vi "TargetCorrection.vi"(8 "error in (no error)":errorcluster, 9 "orientation":dbl, 10 "position(x,y)":dbl[](array[numeric]), 11 "KickToPassReceiverTactic in":refnum<class "KickToPassReceiverTactic.lvclass">) -> (0 "error out":errorcluster, 2 "TargetCorrection":dbl[](array[numeric]), 3 "KickToPassReceiverTactic out":refnum<class "KickToPassReceiverTactic.lvclass">)   [LabVIEW 2021, in "KickToPassReceiverTactic.lvclass"]
uses:
  KickToPassReceiverTactic.lvclass
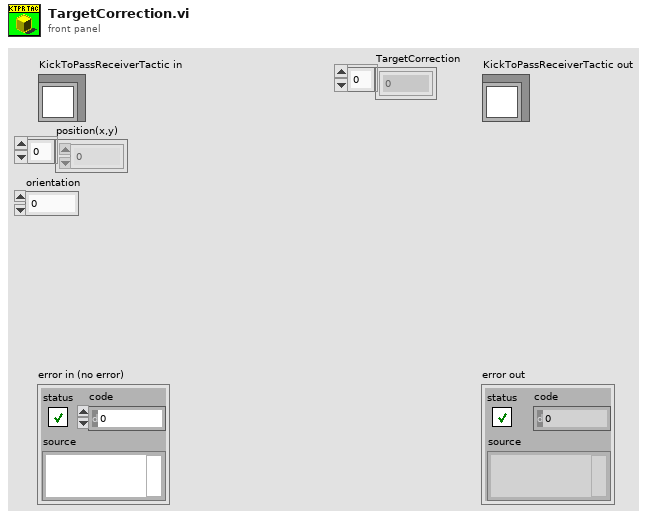
[diagram p1: front panel]
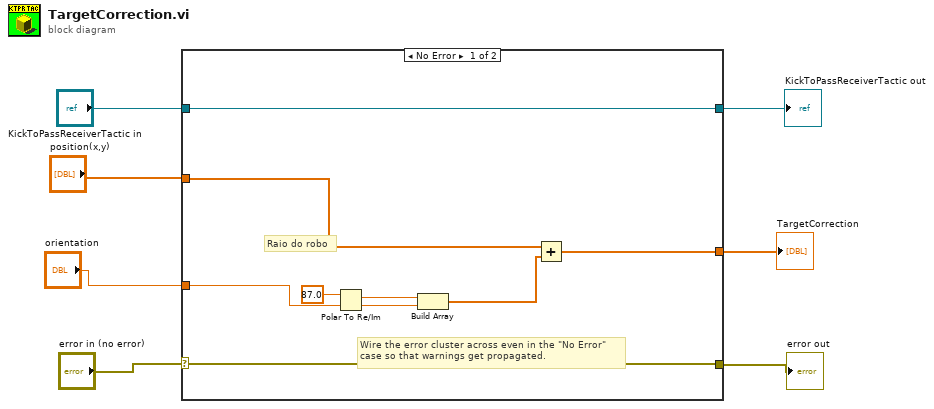
[diagram p0: block diagram]
diagram:
  n1 = case shown="No Error" "error in (no error)" {
    selector: "error in (no error)" -> [w15 w18]
    tunnel: [w15 w18] -> w6
    tunnel: [w16 w17] -> w4
    tunnel: "KickToPassReceiverTactic in" -> [w16 w17]
    tunnel: "position(x,y)" -> [w12 _]
    tunnel: "orientation" -> [w14 _]
    tunnel: [w8 _] -> w1
    frame No Error {
      # "Raio do robo"
      # "Wire the error cluster across even in the \"No Error\"\ncase so that warnings get propagated."
      n2 = Polar To Re/Im(2:w14, 3:87.0 ("r")) -> (0:w10:dbl, 1:w11:dbl)
      n3 = Build Array(w11, w10) -> (w9:dbl[])
      n4 = Add(x=w12, y=w9) -> (x+y=w8:dbl[])
    }
    frame Error {
    }
  }
  "error out" <- w6
  "KickToPassReceiverTactic out" <- w4
  "TargetCorrection" <- w1
